vi "Class Factory.vi"(8 "error in (no error)":errorcluster, 10 "ClassName":string, 11 "FilePath":path) -> (0 "error out":errorcluster, 3 "Instrument":refnum<class "JMETestSolutions.Instrument.lvclass">)   [LabVIEW 2020, in "JMETestSolutions.Instrument.lvlib" / "JMETestSolutions.Instrument.lvclass"]
uses:
  JMETestSolutions.Instrument.lvclass
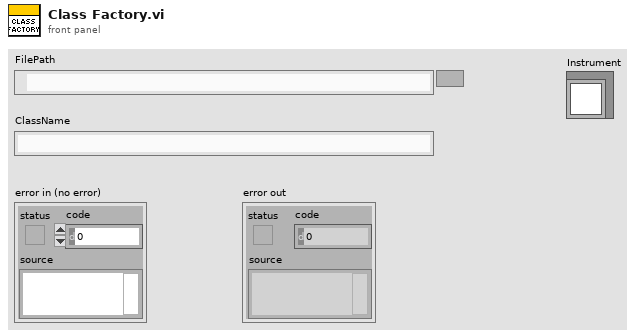
[diagram p1: front panel]
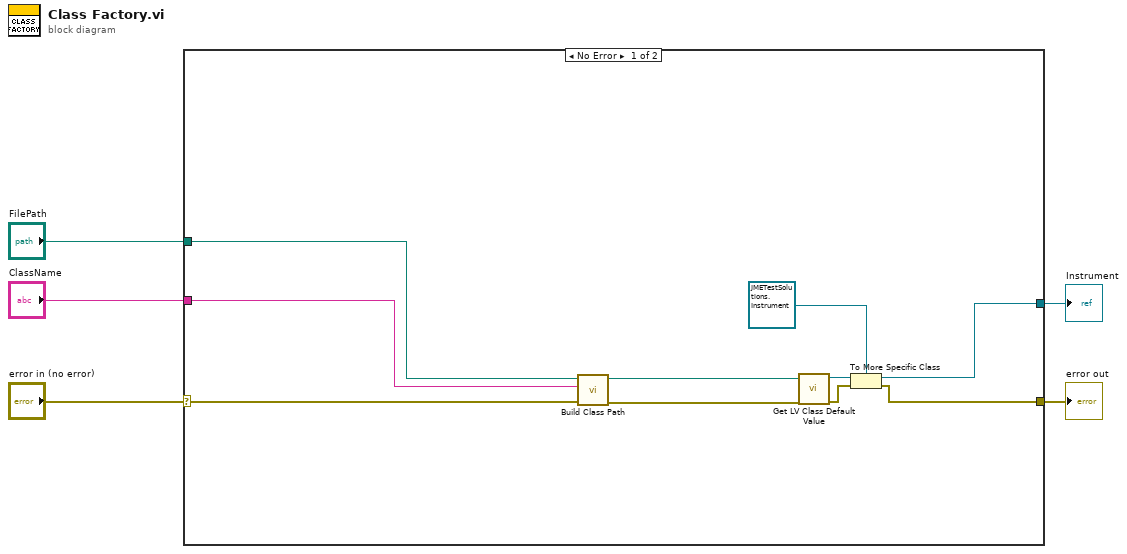
[diagram p0: block diagram]
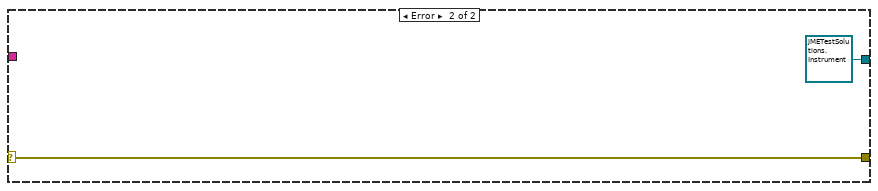
[diagram p2: hidden frame]
diagram:
  n1 = case shown="No Error" "error in (no error)" {
    selector: "error in (no error)" -> [w7 w17]
    tunnel: [w12 w17] -> w4
    tunnel: [w11 refnum<class "JMETestSolutions.Instrument.lvclass"> refnum ("JMETestSolutions.Instrument in")] -> w1
    tunnel: "FilePath" -> [w6 _]
    tunnel: "ClassName" -> [w8 _]
    frame No Error {
      n2 = call "Build Class Path.vi"("Error In"=w7, "Class Name"=w8, "Class Relative Path"=w6) -> ("Error Out"=w9:errorcluster, "Class Path"=w10:path)  [unwired: 7 in]
      n3 = call <vilib>:"Get LV Class Default Value.vi"("error in (no error)"=w9, "class path"=w10) -> ("error out"=w13:errorcluster, "object"=w15:refnum<class>)  [unwired: 8 in]
      n4 = To More Specific Class(target class=refnum<class "JMETestSolutions.Instrument.lvclass"> refnum ("JMETestSolutions.Instrument in"), reference=w15, error in=w13) -> (specific class reference=w11:refnum<class "JMETestSolutions.Instrument.lvclass">, error out=w12:errorcluster)
    }
    frame Error {
    }
  }
  "error out" <- w4
  "Instrument" <- w1
